vi "minutes_to_delay.vi"(6 "already done":i32, 8 "remainder":i32, 9 "selected":bool, 10 "Knob in":refnum<vi>, 11 "delay minutes":i32) -> ()   [LabVIEW 2015]
uses:
  global_stop_calibration.vi
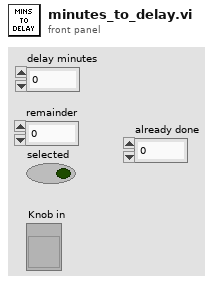
[diagram p1: front panel]
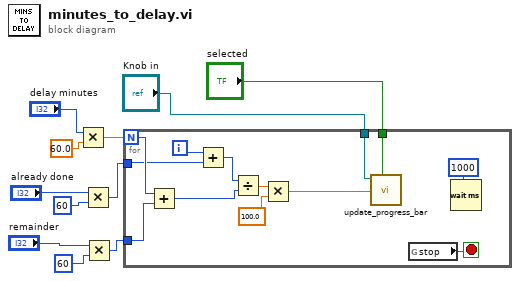
[diagram p0: block diagram]
diagram:
  n1 = Multiply(x="delay minutes", y=60.0) -> (x*y=w9:dbl)
  n2 = Multiply(x="already done", y=60) -> (x*y=w1:i32)
  n3 = Multiply(x="remainder", y=60) -> (x*y=w7:i32)
  n4 = for {
    N: w9 -> [w19]
    tunnel: w7 -> [w17]
    tunnel: "Knob in" -> [w16]
    tunnel: "selected" -> [w15]
    tunnel: w1 -> [w12]
    i -> [w14]
    stop <- w24 stop-if-true
    n5 = Add(x=w19, y=w17) -> (x+y=w18:i32)
    n6 = Add(x=w14, y=w12) -> (x+y=w13:i32)
    n7 = Divide(x=w13, y=w18) -> (x/y=w22:dbl)
    n8 = Multiply(x=w22, y=100.0) -> (x*y=w20:dbl)
    n9 = call "update_progress_bar.vi"("selected"=w15, "Numeric"=w20, "Knob in"=w16) -> ()  [unwired: 8 in, 1 out]
    n10 = global read "global_stop_calibration.vi" "stop"() -> (w24:bool)
    n11 = Wait (ms)(milliseconds to wait=u32 1000) -> ()  [unwired: 1 out]
  }
